vi "Interpret Driver Controls.vi"() -> ()   [LabVIEW 2018]
uses:
  SubSystems/Controllers/Manipulator Controlller/Manipulator Controller Global.vi
  SubSystems/Lift/Lift Global.vi
  SubSystems/Controllers/Driver Controller/Driver Controller Global.vi
  SubSystems/Cargo Intake/Cargo Intake Global.vi
  SubSystems/Drive Train/Drive Train Global.vi
  SubSystems/Hatch Panel Intake/Hatch Panel Intake Global.vi
panel:
  in  "y":dbl=0.6 format="%#_13g"
  in  "Y Slower":dbl=0.65
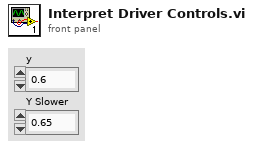
[diagram p1: front panel]
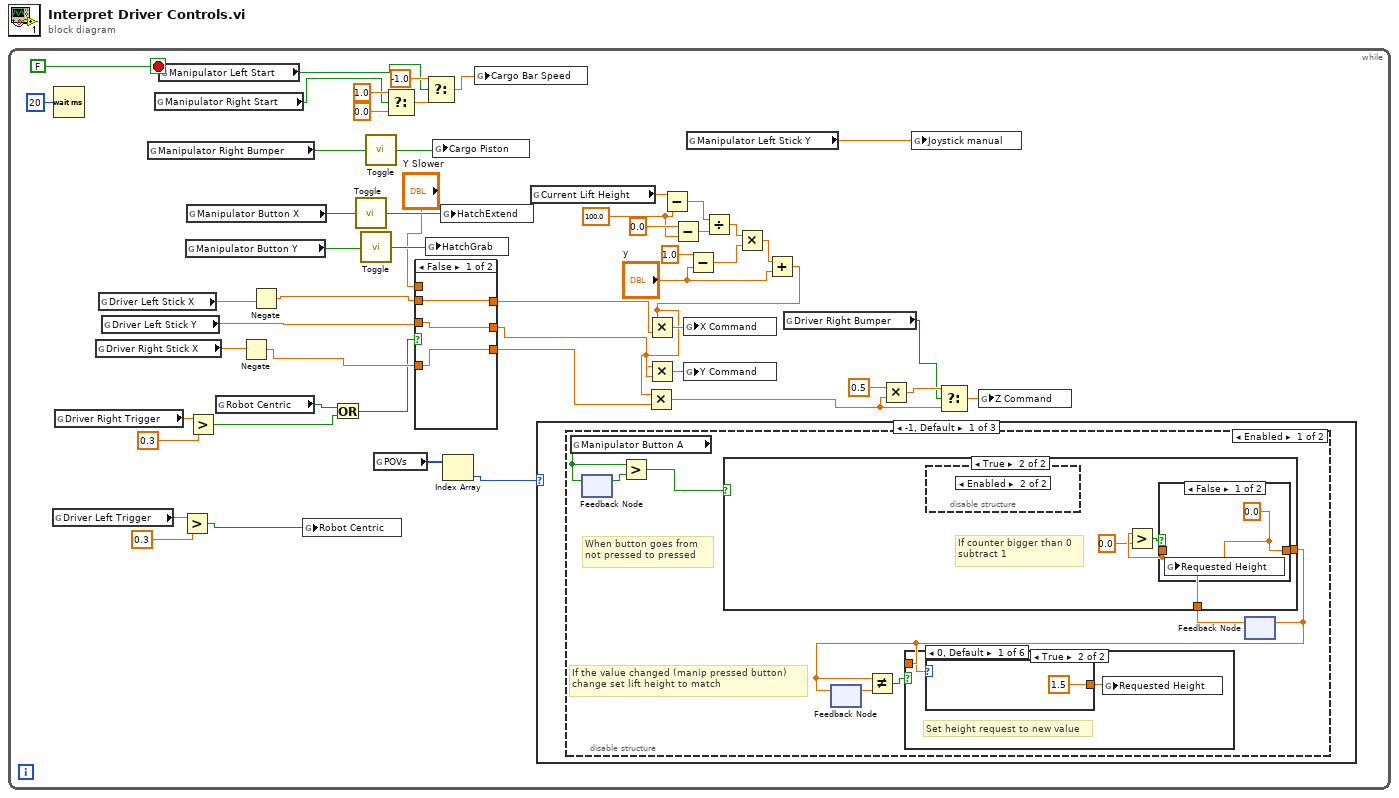
[diagram p0: block diagram]
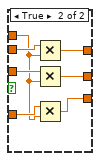
[diagram p2: hidden frame]
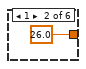
[diagram p4: hidden frame]
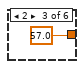
[diagram p5: hidden frame]
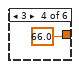
[diagram p6: hidden frame]
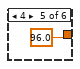
[diagram p7: hidden frame]
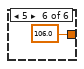
[diagram p8: hidden frame]
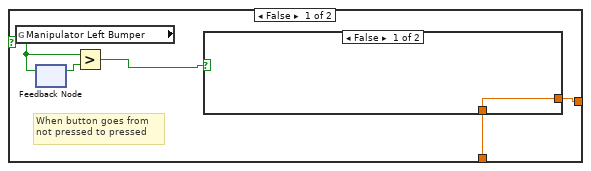
[diagram p9: hidden frame]
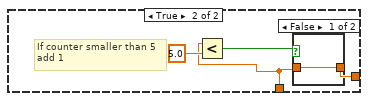
[diagram p10: hidden frame]
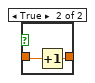
[diagram p11: hidden frame]
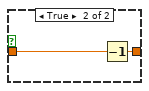
[diagram p12: hidden frame]
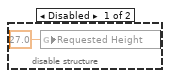
[diagram p13: hidden frame]
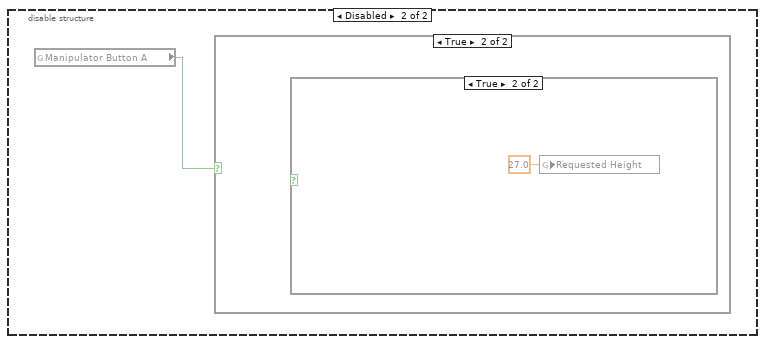
[diagram p14: hidden frame]
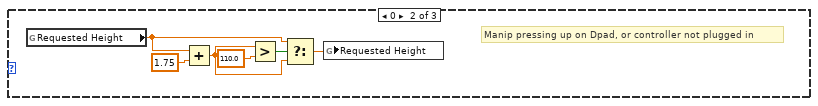
[diagram p17: hidden frame]
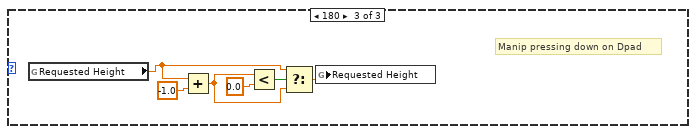
[diagram p18: hidden frame]
diagram:
  n1 = while {
    stop <- FALSE stop-if-true
    w15 = 100.0 ("y")
    n2 = global read "Driver Controller Global.vi" "Driver Left Trigger"() -> (w10:dbl)
    n3 = Wait (ms)(milliseconds to wait=u32 20) -> ()  [unwired: 1 out]
    n4 = global read "Driver Controller Global.vi" "Driver Right Trigger"() -> (w35:dbl)
    n5 = global read "Driver Controller Global.vi" "Driver Right Stick X"() -> (w41:dbl)
    n6 = global read "Driver Controller Global.vi" "Driver Left Stick X"() -> (w42:dbl)
    n7 = global read "Driver Controller Global.vi" "Driver Left Stick Y"() -> (w13:dbl)
    n8 = global read "Manipulator Controller Global.vi" "Manipulator Right Bumper"() -> (w36:bool)
    n9 = global read "Manipulator Controller Global.vi" "Manipulator Right Start"() -> (w44:bool)
    n10 = global read "Manipulator Controller Global.vi" "Manipulator Left Start"() -> (w45:bool)
    n11 = Greater?(x=w10, y=0.3) -> (0:w5:bool)
    n12 = global read "Manipulator Controller Global.vi" "Manipulator Button Y"() -> (w40:bool)
    n13 = global read "Manipulator Controller Global.vi" "Manipulator Button X"() -> (w51:bool)
    n14 = Greater?(x=w35, y=0.3) -> (0:w3:bool)
    n15 = global read "Drive Train Global.vi" "Robot Centric"() -> (w2:bool)
    n16 = Negate(x=w41) -> (-x=w12:dbl)
    n17 = Negate(x=w42) -> (-x=w14:dbl)
    n18 = global write "Drive Train Global.vi" "Robot Centric"(w5) -> ()
    n19 = Or(x=w2, y=w3) -> (x .or. y?=w1:bool)
    n20 = call "Toggle.vi"("Input"=w51) -> ("Output"=w50:bool)
    n21 = call "Toggle.vi"("Input"=w40) -> ("Output"=w39:bool)
    n22 = call "Toggle.vi"("Input"=w36) -> ("Output"=w37:bool)
    n23 = global read "Manipulator Controller Global.vi" "POVs"() -> (w33:i16[])
    n24 = Select(t=1.0, s=w44, f=0.0) -> (s? t:f=w49:dbl)
    n25 = case shown="False" w1 {
      tunnel: w14 -> [w56 w63]
      tunnel: "Y Slower" -> [_ w57]
      tunnel: [w56 w62] -> w28
      tunnel: [w55 w61] -> w27
      tunnel: [w54 w60] -> w26
      tunnel: w13 -> [w55 w59]
      tunnel: w12 -> [w54 w58]
      frame False {
      }
      frame True {
        n26 = Multiply(x=w63, y=w57) -> (x*y=w62:dbl)
        n27 = Multiply(x=w59, y=w57) -> (x*y=w61:dbl)
        n28 = Multiply(x=w58, y=w57) -> (x*y=w60:dbl)
      }
    }
    n29 = Select(t=-1.0, s=w45, f=w49) -> (s? t:f=w43:dbl)
    n30 = global write "Hatch Panel Intake Global.vi" "HatchGrab"(w39) -> ()
    n31 = global write "Cargo Intake Global.vi" "Cargo Piston"(w37) -> ()
    n32 = global write "Hatch Panel Intake Global.vi" "HatchExtend"(w50) -> ()
    n33 = Index Array(array=w33) -> (element=w32:i16)  [unwired: 1 in]
    n34 = global write "Cargo Intake Global.vi" "Cargo Bar Speed"(w43) -> ()
    n35 = global read "Lift Global.vi" "Current Lift Height"() -> (w25:dbl)
    n36 = case shown="-1, Default" w32 {
      frame -1, Default {
        n37 = disable-structure shown="Enabled" {
          frame Enabled {
            # "If the value changed (manip pressed button)\nchange set lift height to match"
            # "When button goes from\nnot pressed to pressed"
            n38 = global read "Manipulator Controller Global.vi" "Manipulator Button A"() -> (w69:bool)
            n39 = feedback #1() -> (w70:bool)  [unwired: 1 in]
            n40 = feedback-in #1(w69) -> ()
            n41 = Greater?(x=w69, y=w70) -> (0:w64:bool)
            n42 = feedback #2() -> (w67:dbl)  [unwired: 1 in]
            n43 = feedback #3() -> (w68:dbl)  [unwired: 1 in]
            n44 = case shown="True" w64 {
              tunnel: [w80 w95] -> w66
              tunnel: w68 -> [w81 w94]
              frame False {
                # "When button goes from\nnot pressed to pressed"
                n45 = global read "Manipulator Controller Global.vi" "Manipulator Left Bumper"() -> (w83:bool)
                n46 = feedback #4() -> (w82:bool)  [unwired: 1 in]
                n47 = feedback-in #4(w83) -> ()
                n48 = Greater?(x=w83, y=w82) -> (0:w79:bool)
                n49 = case shown="False" w79 {
                  tunnel: w81 -> [w84 w86]
                  tunnel: [w84 w88] -> w80
                  frame False {
                  }
                  frame True {
                    # "If counter smaller than 5\nadd 1"
                    n50 = Less?(x=w86, y=5.0) -> (x < y?=w85:bool)
                    n51 = case shown="False" w85 {
                      tunnel: [w89 w91] -> w88
                      tunnel: w86 -> [w89 w90]
                      frame False {
                      }
                      frame True {
                        n52 = Increment(x=w90) -> (x+1=w91:dbl)
                      }
                    }
                  }
                }
              }
              frame True {
                # "If counter bigger than 0\nsubtract 1"
                n53 = disable-structure shown="Enabled" {
                  frame Disabled {
                    n54 = global write "Lift Global.vi" "Requested Height"(27.0 ("Requested Height")) -> ()
                  }
                  frame Enabled {
                  }
                }
                n55 = Greater?(x=w94, y=0.0) -> (0:w93:bool)
                n56 = case shown="False" w93 {
                  tunnel: [w96 w98] -> w95
                  tunnel: w94 -> [_ w97]
                  frame False {
                    w96 = 0.0 ("y")
                    n57 = global write "Lift Global.vi" "Requested Height"(w96) -> ()
                  }
                  frame True {
                    n58 = Decrement(x=w97) -> (x-1=w98:dbl)
                  }
                }
              }
            }
            n59 = feedback-in #2(w66) -> ()
            n60 = Not Equal?(x=w66, y=w67) -> (x != y?=w65:bool)
            n61 = case shown="True" w65 {
              tunnel: w66 -> [_ w71]
              frame False {
                # "Manipulator didnt request change"
              }
              frame True {
                # "Set height request to new value"
                n62 = case shown="0, Default" w71 {
                  tunnel: [1.5 ("Requested Height") 26.0 ("Requested Height") 57.0 ("Requested Height") 66.0 ("Requested Height") 96.0 ("Requested Height") 106.0 ("Requested Height")] -> w72
                  frame 0, Default {
                  }
                  frame 1 {
                  }
                  frame 2 {
                  }
                  frame 3 {
                  }
                  frame 4 {
                  }
                  frame 5 {
                  }
                }
                n63 = global write "Lift Global.vi" "Requested Height"(w72) -> ()
              }
            }
            n64 = feedback-in #3(w66) -> ()
          }
          frame Disabled {
            n65 = global read "Manipulator Controller Global.vi" "Manipulator Button A"() -> (w100:bool)
            n66 = case shown="True" w100 {
              frame False {
              }
              frame True {
                n67 = case shown="True" {
                  selector: _ -> [_ _]
                  frame False {
                  }
                  frame True {
                    n68 = global write "Lift Global.vi" "Requested Height"(27.0 ("Requested Height")) -> ()
                  }
                }
              }
            }
          }
        }
      }
      frame 0 {
        # "Manip pressing up on Dpad, or controller not plugged in"
        n69 = global read "Lift Global.vi" "Requested Height"() -> (w103:dbl)
        n70 = Add(x=w103, y=1.75) -> (x+y=w102:dbl)
        n71 = Greater?(x=w102, y=110.0) -> (0:w104:bool)
        n72 = Select(t=w103, s=w104, f=w102) -> (s? t:f=w105:dbl)
        n73 = global write "Lift Global.vi" "Requested Height"(w105) -> ()
      }
      frame 180 {
        # "Manip pressing down on Dpad"
        n74 = global read "Lift Global.vi" "Requested Height"() -> (w108:dbl)
        n75 = Add(x=w108, y=-1.0) -> (x+y=w110:dbl)
        n76 = Less?(x=w110, y=0.0) -> (x < y?=w111:bool)
        n77 = Select(t=w108, s=w111, f=w110) -> (s? t:f=w109:dbl)
        n78 = global write "Lift Global.vi" "Requested Height"(w109) -> ()
      }
    }
    n79 = Subtract(x=w25, y=w15) -> (x-y=w24:dbl)
    n80 = Subtract(x=0.0 ("y"), y=w15) -> (x-y=w23:dbl)
    n81 = global read "Manipulator Controller Global.vi" "Manipulator Left Stick Y"() -> (w38:dbl)
    n82 = Subtract(x=1.0 ("y"), y="y") -> (x-y=w20:dbl)
    n83 = Divide(x=w24, y=w23) -> (x/y=w21:dbl)
    n84 = Multiply(x=w21, y=w20) -> (x*y=w19:dbl)
    n85 = Add(x=w19, y="y") -> (x+y=w17:dbl)
    n86 = Multiply(x=w17, y=w26) -> (x*y=w8:dbl)
    n87 = Multiply(x=w17, y=w28) -> (x*y=w30:dbl)
    n88 = Multiply(x=w17, y=w27) -> (x*y=w29:dbl)
    n89 = global write "Drive Train Global.vi" "X Command"(w30) -> ()
    n90 = global write "Drive Train Global.vi" "Y Command"(w29) -> ()
    n91 = global read "Driver Controller Global.vi" "Driver Right Bumper"() -> (w4:bool)
    n92 = Multiply(x=0.5, y=w8) -> (x*y=w7:dbl)
    n93 = global write "Lift Global.vi" "Joystick manual"(w38) -> ()
    n94 = Select(t=w7, s=w4, f=w8) -> (s? t:f=w9:dbl)
    n95 = global write "Drive Train Global.vi" "Z Command"(w9) -> ()
  }
